vi "SEQ Preview Queue.vi"(8 "error in":errorcluster) -> (0 "error out":errorcluster, 3 "SEQ Data":T1)   [LabVIEW 2019, in "sbRIO9623.lvlib"]
uses:
  sbRIO9623.lvlib
  SEQ Data.ctl
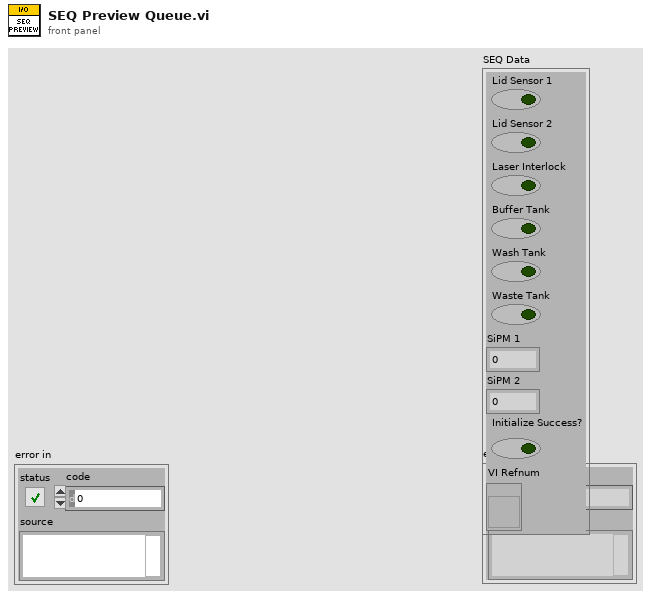
[diagram p1: front panel]
types:
  T1 = typedef "sbRIO9623.lvlib/SEQ Data.ctl" = cluster{"Lid Sensor 1":bool, "Lid Sensor 2":bool, "Laser Interlock":bool, "Buffer Tank":bool, "Wash Tank":bool, "Waste Tank":bool, "SiPM 1":fxp<+,20,5>, "SiPM 2":fxp<+,20,5>, "Initialize Success?":bool, "VI Refnum":refnum<vi>}
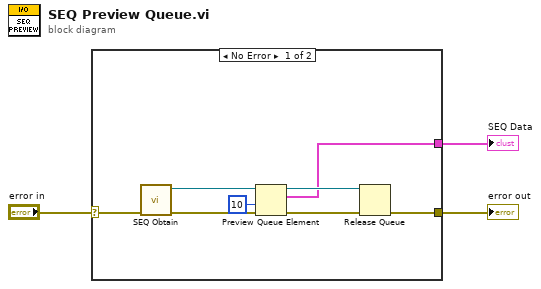
[diagram p0: block diagram]
diagram:
  n1 = case shown="No Error" "error in" {
    selector: "error in" -> [w7 w12]
    tunnel: [w8 w12] -> w2
    tunnel: [w4 _] -> w1
    frame No Error {
      n2 = call "SEQ Obtain.vi"("error in"=w7) -> ("error out"=w6:errorcluster, "queue out"=w5:refnum<queue>)  [unwired: 9 in]
      n3 = Preview Queue Element(queue=w5, timeout in ms (-1)=10, error in (no error)=w6) -> (queue out=w9:refnum<queue>, element=w4:T1, error out=w10:errorcluster)  [unwired: 1 out]
      n4 = Release Queue(queue=w9, error in (no error)=w10) -> (error out=w8:errorcluster)  [unwired: 1 in, 2 out]
    }
    frame Error {
    }
  }
  "error out" <- w2
  "SEQ Data" <- w1
